vi "Actor Core.vi"(8 "error in":errorcluster, 11 "Customer With Cell Phone in":refnum<class "Customer With Cell Phone.lvclass">) -> (0 "error out":errorcluster, 3 "Actor out":refnum<class "Actor.lvclass">)   [LabVIEW 2023, in "Customer With Cell Phone.lvlib" / "Customer With Cell Phone.lvclass"]
doc: "(<B>Filename</B>: Actor Framework.lvlib:Actor.lvclass:Actor Core.vi)\n\nReceives messages to the actor, reacts to them, and initiates any error handling that may shut the actor down.\n\nDescendant classes may override this VI to append parallel tasks for the actor to complete while it handles messages. Overrides use the Call Parent Method node."
uses:
  Customer With Cell Phone.lvclass
  c:/dev/_r/4/eng/lv-core/lvpostprocessingd/lv_mc_x86_64/dist_i386/vi.lib/ActorFramework/Actor/Actor.lvclass
  <vilib>/ActorFramework/Actor/Actor.lvclass
  <vilib>/ActorFramework/Actor/Actor.lvclass/Actor.ctl
  <vilib>/ActorFramework/Message Enqueuer/Message Enqueuer.lvclass/Message Enqueuer.ctl
  Customer With Cell Phone.lvclass/Customer With Cell Phone.ctl
  <vilib>/ActorFramework/Message Enqueuer/Init from Existing Queue.vi
  <vilib>/ActorFramework/Message Enqueuer/Enqueue.vi
  CustomerWithCellPhone Messages/MakeCall Msg/MakeCall Msg.lvclass
  c:/dev/_r/4/eng/lv-core/lvpostprocessingd/lv_mc_x86_64/dist_i386/vi.lib/ActorFramework/Message/Message.lvclass
  <vilib>/ActorFramework/Message Priority Queue/Priority Enqueue.vi
  Customer.lvclass
  <vilib>/ActorFramework/Message Enqueuer/Message Enqueuer.lvclass
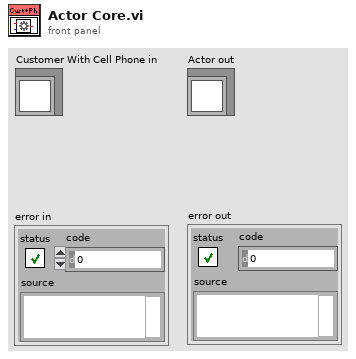
[diagram p1: front panel]
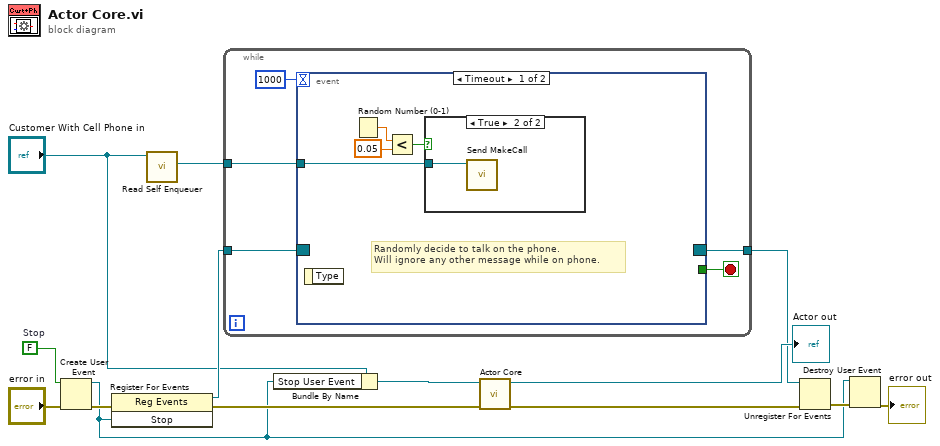
[diagram p0: block diagram]
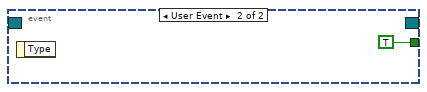
[diagram p3: hidden frame]
diagram:
  w8 = FALSE  # Stop
  n1 = Create User Event(user event datatype=w8, error in="error in") -> (user event=w2:refnum<user-event>, error out=w7:errorcluster)
  n2 = register-events(error in=w7, w2) -> (reference out=w13:refnum<event-registration>, error out=w6:errorcluster)  [unwired: 1 in]
  n3 = call <vilib>:"Read Self Enqueuer.vi"("Actor"="Customer With Cell Phone in") -> ("Self Enqueuer"=w10:refnum<class "Message Enqueuer.lvclass">)  [unwired: 10 in]
  n4 = while {
    tunnel: w13 -> [w18]
    tunnel: [w17] -> w12
    tunnel: w10 -> [w15]
    stop <- w16 stop-if-true
    n5 = event shown="[0] Timeout" {
      selector: w18 -> [_ _]
      dyn-events: [_ _] -> w17
      timeout: 1000 -> [_ _]
      tunnel: [_ TRUE] -> w16
      tunnel: w15 -> [w20 _]
      event Timeout {
        # "Randomly decide to talk on the phone.\nWill ignore any other message while on phone."
        n6 = event-data() -> ()  [unwired: 1 in, 1 out]
        n7 = Random Number (0-1)() -> (number: 0 to 1=w23:dbl)
        n8 = Less?(x=w23, y=0.05) -> (x < y?=w21:bool)
        n9 = case shown="True" w21 {
          tunnel: w20 -> [_ w24]
          frame False {
          }
          frame True {
            n10 = call "Send MakeCall.vi"("Message Enqueuer"=w24) -> ()  [unwired: 9 in, 2 out]
          }
        }
      }
      event User Event {
        n11 = event-data() -> ()  [unwired: 1 in, 1 out]
      }
    }
  }
  n12 = Bundle By Name(cluster="Customer With Cell Phone in", "Stop User Event"=w2) -> (w1:refnum<class "Customer With Cell Phone.lvclass">)
  n13 = call-parent "Actor Core.vi"("error in"=w6, "Customer in"=w1) -> ("error out"=w11:errorcluster, "Actor out"=→"Actor out":refnum<class "Actor.lvclass">)  [unwired: 8 in]
  n14 = Unregister For Events(event registration refnum=w12, error in=w11) -> (error out=w4:errorcluster)
  n15 = Destroy User Event(user event=w2, error in=w4) -> (error out=→"error out":errorcluster)
